vi "Test Validate Loki Json Against Schema.vi"(8 "error in (no error)":errorcluster) -> (0 "error out":errorcluster)   [LabVIEW 2017, in "UT_LokiJsonFormatter.lvlib"]
doc: "Template for an unit test with caraya in the \"Given, When, Then\" structure from James."
uses:
  UT_LokiJsonFormatter.lvlib
  Source/HSE-Logger/LogLevel.ctl
  <vilib>/addons/_JKI Toolkits/Caraya/classes/Assert/Assert False.vi
  <vilib>/addons/_JKI Toolkits/Caraya/classes/Test/Test.lvclass
  <vilib>/addons/_JKI Toolkits/Caraya/classes/Assert/Assert.lvclass
  Source/HSE-Logger/Formatter/LokiJsonFormatter/LokiJsonFormatter.lvclass
  <vilib>/JDP Science/JSONtext/JSONtext.lvlib
  Source/HSE-Logger/LogRecord/LogRecord.lvclass
  Source/HSE-Logger/hse-logger.lvlib
panel:
  # "Connector Pane"
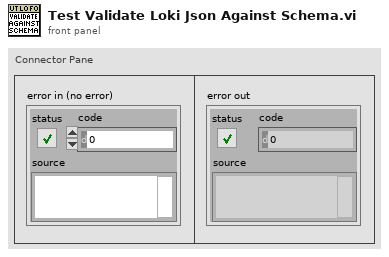
[diagram p1: front panel]
types:
  T1 = typedef "hse-logger.lvlib/LogLevel.ctl" = enum16{"DEBUG", "INFO", "WARNING", "ERROR", "CRITICAL"}
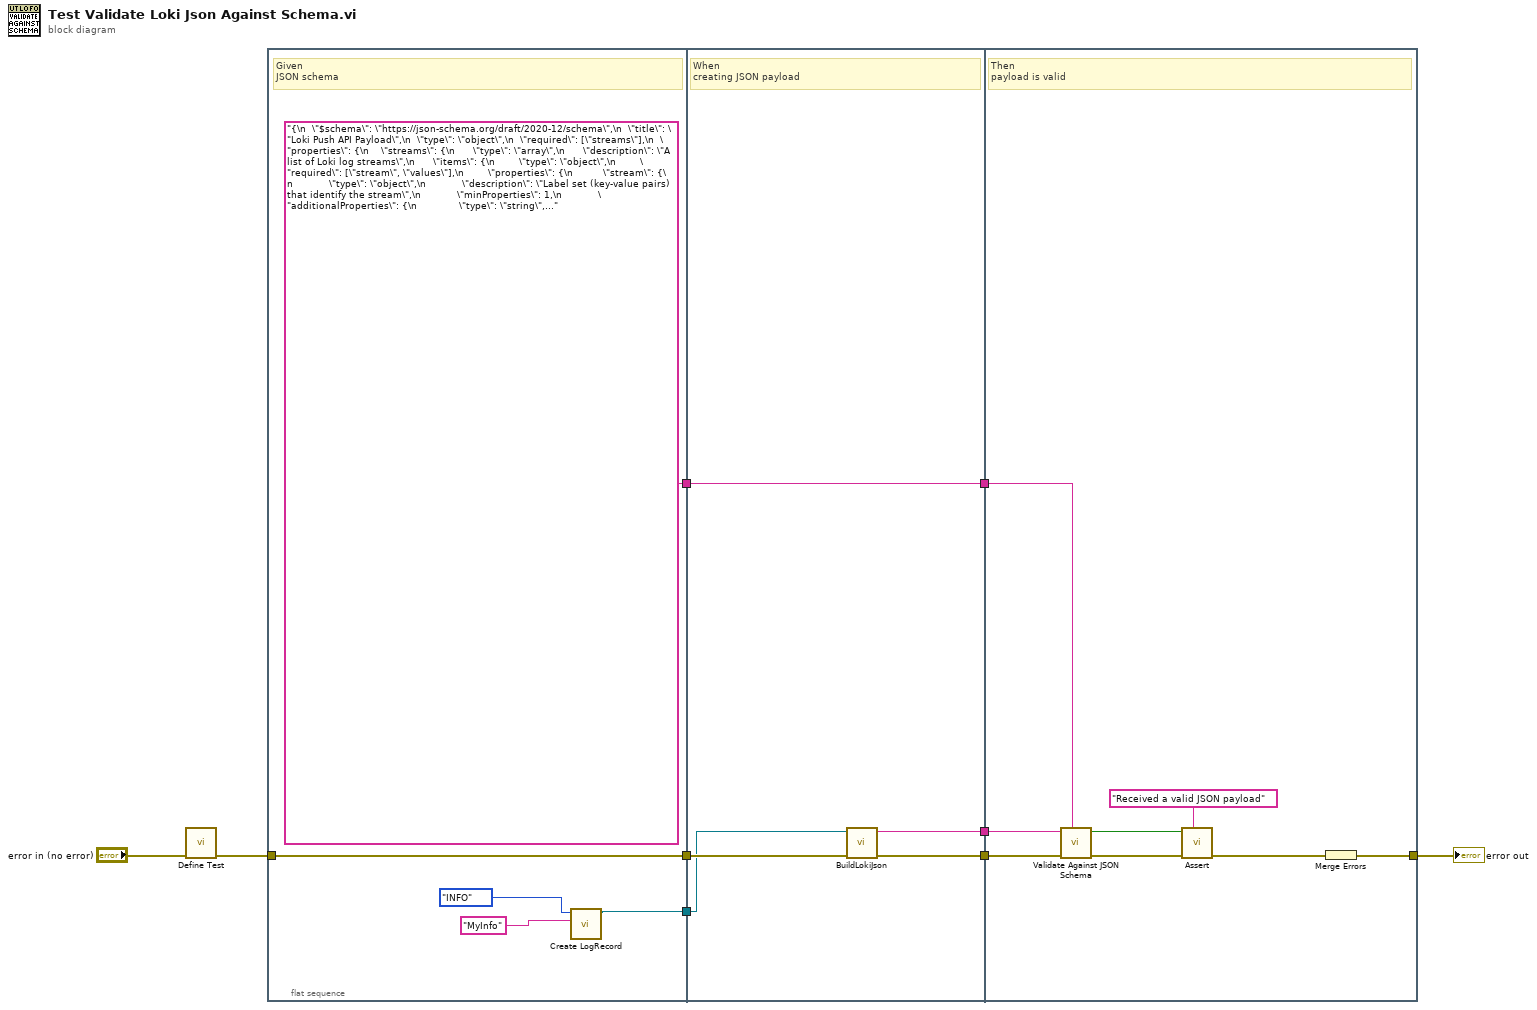
[diagram p0: block diagram]
diagram:
  n1 = call <vilib>:"Define Test.vi"("error in (no error)"="error in (no error)") -> ("error out"=w6:errorcluster)  [unwired: 9 in, 1 out]
  n2 = flat-sequence {
    tunnel: w6 -> [w14]
    tunnel: [w14] -> w9
    tunnel: ["{\n  \"$schema\": \"https://json-schema.org/draft/2020-12/schema\",\n  \"title\": \"Loki Push API Payload\",\n  \"type\": \"object\",\n  \"required\": [\"streams\"],\n  \"properties\": {\n    \"streams\": {\n      \"type\": \"array\",\n      \"description\": \"A list of Loki log streams\",\n      \"items\": {\n        \"type\": \"object\",\n        \"required\": [\"stream\", \"values\"],\n        \"properties\": {\n          \"stream\": {\n            \"type\": \"object\",\n            \"description\": \"Label set (key-value pairs) that identify the stream\",\n            \"minProperties\": 1,\n            \"additionalProperties\": {\n              \"type\": \"string\",\n              \"description\": \"Label values must be strings\"\n            }\n          },\n          \"values\": {\n            \"type\": \"array\",\n            \"description\": \"List of log entries for this stream\",\n            \"items\": {\n              \"type\": \"array\",\n              \"description\": \"A log entry: [timestamp, line]\",\n              \"prefixItems\": [\n                {\n                  \"type\": \"string\",\n                  \"pattern\": \"^[0-9]+$\",\n                  \"description\": \"Unix timestamp in nanoseconds, as a string\"\n                },\n                {\n                  \"type\": \"string\",\n                  \"description\": \"Log message line\"\n                }\n              ],\n              \"minItems\": 2,\n              \"maxItems\": 2\n            }\n          }\n        }\n      }\n    }\n  }\n}" ("JSON Schema")] -> w3
    tunnel: [w12] -> w1
    tunnel: w9 -> [w18]
    tunnel: [w19] -> w5
    tunnel: [w17] -> w4
    tunnel: w3 -> [w16]
    tunnel: [w16] -> w2
    tunnel: w1 -> [w15]
    tunnel: [w26] -> w8
    tunnel: w5 -> [w23]
    tunnel: w4 -> [w22]
    tunnel: w2 -> [w21]
    frame #0 {
      # "Given\nJSON schema"
      n3 = call "Create LogRecord.vi"("Message"="MyInfo", "Level"=LogLevel."INFO") -> ("LogRecord out"=w12:refnum<class "LogRecord.lvclass">)  [unwired: 8 in, 1 out]
    }
    frame #1 {
      # "When\ncreating JSON payload"
      n4 = call "BuildLokiJson.vi"("error in (no error)"=w18, "LogRecord"=w15) -> ("error out"=w19:errorcluster, "<JSON> out"=w17:string)  [unwired: 8 in]
    }
    frame #2 {
      # "Then\npayload is valid"
      n5 = call <vilib>:"Validate Against JSON Schema.vi"("JSON Schema"=w21, "error in (no error)"=w23, "JSON"=w22) -> ("error out"=w24:errorcluster, "Invalid"=w20:bool)  [unwired: 4 in, 3 out]
      n6 = call-poly <vilib>:"Assert.vi"("Label"="Received a valid JSON payload", "error in (no error)"=w24, "False?"=w20) -> ("error out"=w27:errorcluster)  [unwired: 7 in, 1 out]
      n7 = Merge Errors(w27) -> (w26:errorcluster)
    }
  }
  "error out" <- w8
